vi "Configure TS Results.vi"(8 "error in":errorcluster, 11 "Test Stand in":refnum<class "Generic Test Stand.lvclass">) -> (0 "error out":errorcluster, 3 "Test Stand out":refnum<class "Generic Test Stand.lvclass">)   [LabVIEW 2019, in "Generic Test Stand.lvclass"]
uses:
  Generic Test Stand.lvclass
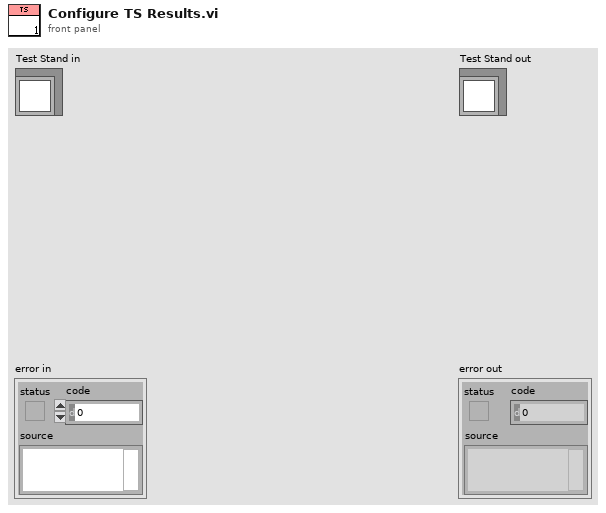
[diagram p1: front panel]
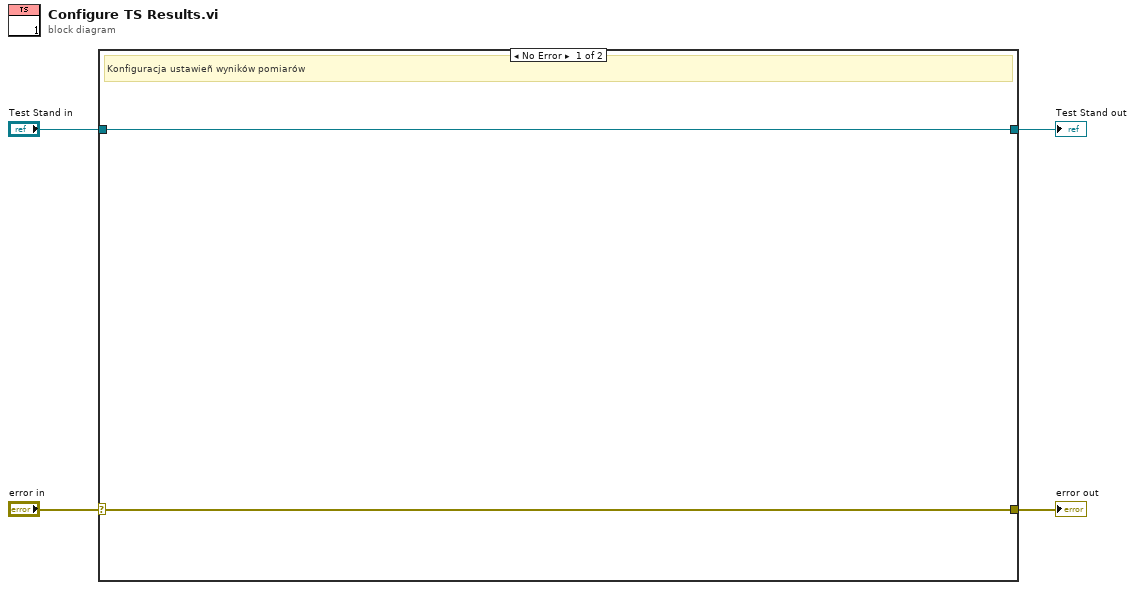
[diagram p0: block diagram]
diagram:
  n1 = case shown="No Error" "error in" {
    selector: "error in" -> [w5 w8]
    tunnel: "Test Stand in" -> [w6 w7]
    tunnel: [w6 w7] -> w3
    tunnel: [w5 w8] -> w1
    frame No Error {
      # "Konfiguracja ustawieñ wyników pomiarów"
    }
    frame Error {
    }
  }
  "error out" <- w1
  "Test Stand out" <- w3
